vi "main_T.vi"() -> ()   [LabVIEW 2017]
uses:
  <vilib>/Platform/TimedLoop/XDataNode/timing_clust.ctl
  <vilib>/Platform/TimedLoop/XDataNode/nitl_modes.ctl
  <vilib>/Platform/TimedLoop/XDataNode/wakeup.ctl
  <vilib>/platform/TimedLoop/XDataNode/XDataNode.xnode
  <vilib>/Platform/TimedLoop/XDataNode/XDNodeRunTimeDep.lvlib
panel:
  out "Alarm Status":bool
  out "dt (ms)":u32
  in  "Tab Control":enum32{"Page 1", "Page 2"}(tab)
  in  "Pause Button 4":bool
  in  "Pause Button 3":bool
  in  "Pause Button 2":bool
  in  "Pause Button":bool
  in  "save RPM as excel":bool
  in  "save RPM as image":bool
  in  "save torque as excel":bool
  in  "save torque as image":bool
  in  "save flow as excel":bool
  in  "save flow as image":bool
  in  "save pressure as excel":bool
  in  "save press as image":bool
  out "RPM Graph":cluster{dbl[], dbl[]}(graph)
  out "t (sec)":dbl format="%#.3f"
  out "dt (sec)":dbl format="%#.3f"
  out "Torque Graph":cluster{dbl[], dbl[]}(graph)
  out "Flow Graph":cluster{dbl[], dbl[]}(graph)
  out "NI1":tag caption="NI device"
  out "Pressure Graph":cluster{dbl[], dbl[]}(graph)
  out "Turbine RPM":dbl format="%#.3f"
  out "Torque [N.m]":dbl format="%#.3f"
  out "Flow [L/min]":dbl format="%#.3f"
  out "Pressure [bar]":dbl format="%#.3f"
  out "Alarm":bool
  out "ON/OFF Pump":bool
  out "Ready / Not ready":bool
  in  "Exit":bool
  in  "Reset Chart":bool
  # "Turbine Training Unit"
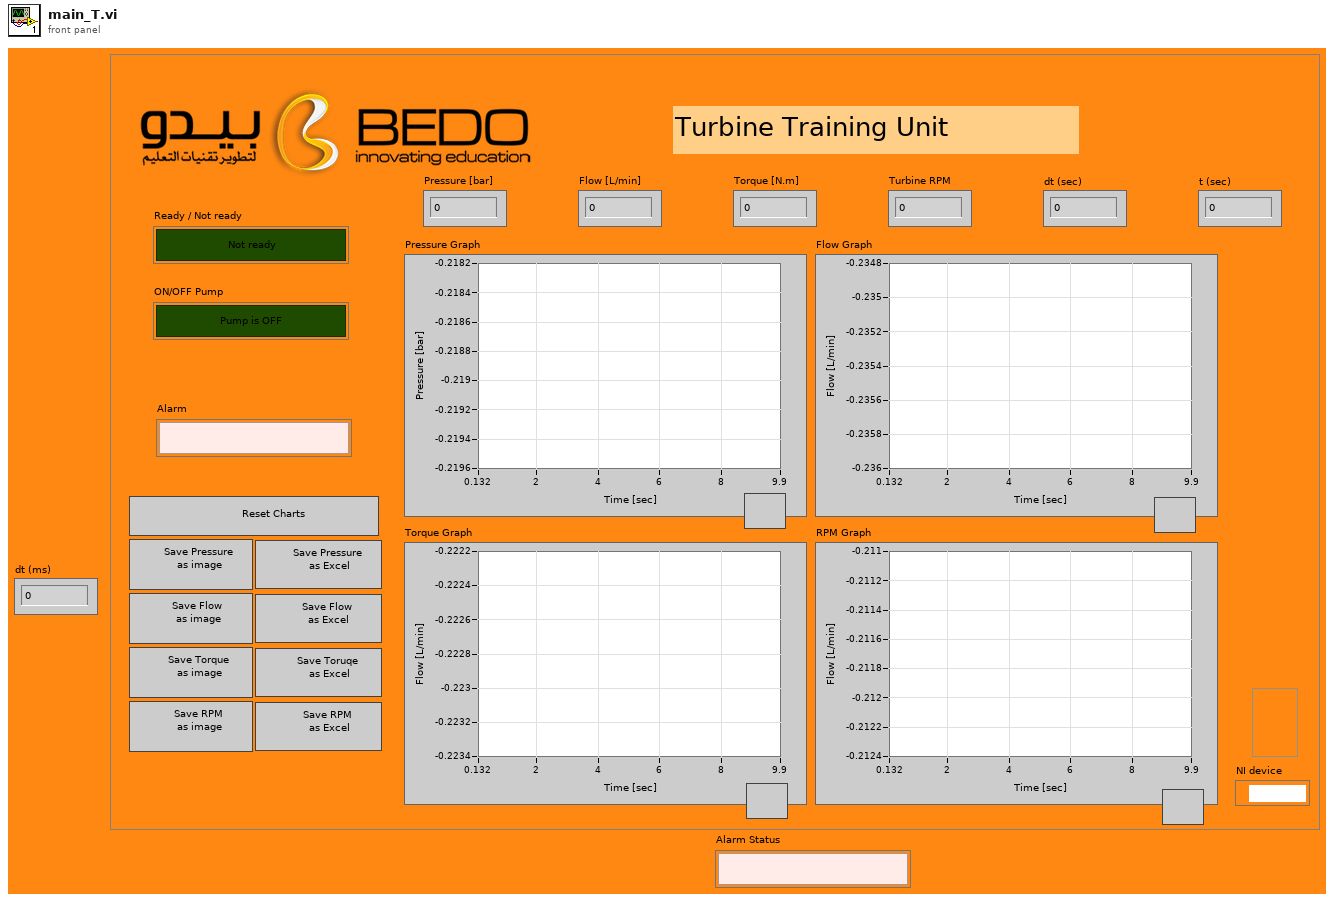
[diagram p1: front panel]
types:
  T1 = enum32{"Invalid", "Standard", "Closed", "Hidden", "Minimized", "Maximized"}
  T2 = typedef "XDNodeRunTimeDep.lvlib/timing_clust.ctl" = cluster{"Expected End [f-1]":u64, "Actual End [f-1]":u64, "Finished Late? [f-1]":bool, "Expected End [i-1]":u64, "Actual End [i-1]":u64, "Finished Late? [i-1]":bool, "Expected Start [i]":u64, "Actual Start [i]":u64, "Expected Start [f]":u64, "Actual Start [f]":u64, "Source Name":string, "Structure Name":string, "Period":i64, "Deadline":i64, "Offset":i64, "Start":i64, "Priority":i32, "Timeout":i32, "Mode":T3, "Wakeup Reason":T4, "Error":errorcluster, "Source Type":string, "Secondary Source Type":string, "Global End Time":u64, "Global Start Time":u64, "Frame Duration":u64, "Iteration Duration":u64, "Assigned CPU":i32, "I/O Scan Engine Mode":u32}
  T3 = typedef "XDNodeRunTimeDep.lvlib/nitl_modes.ctl" = enum32{"No Change", "Process missed periods, maintain original phase", "Discard missed periods, maintain original phase", "Process missed periods, ignore original phase", "Discard missed periods, ignore original phase"}
  T4 = typedef "XDNodeRunTimeDep.lvlib/wakeup.ctl" = enum32{"Normal", "Aborted", "Asynchronous wakeup", "Timing source error", "Timed loop error", "Timeout"}
  T5 = typedef "Sound Output Task ID.ctl" = u32
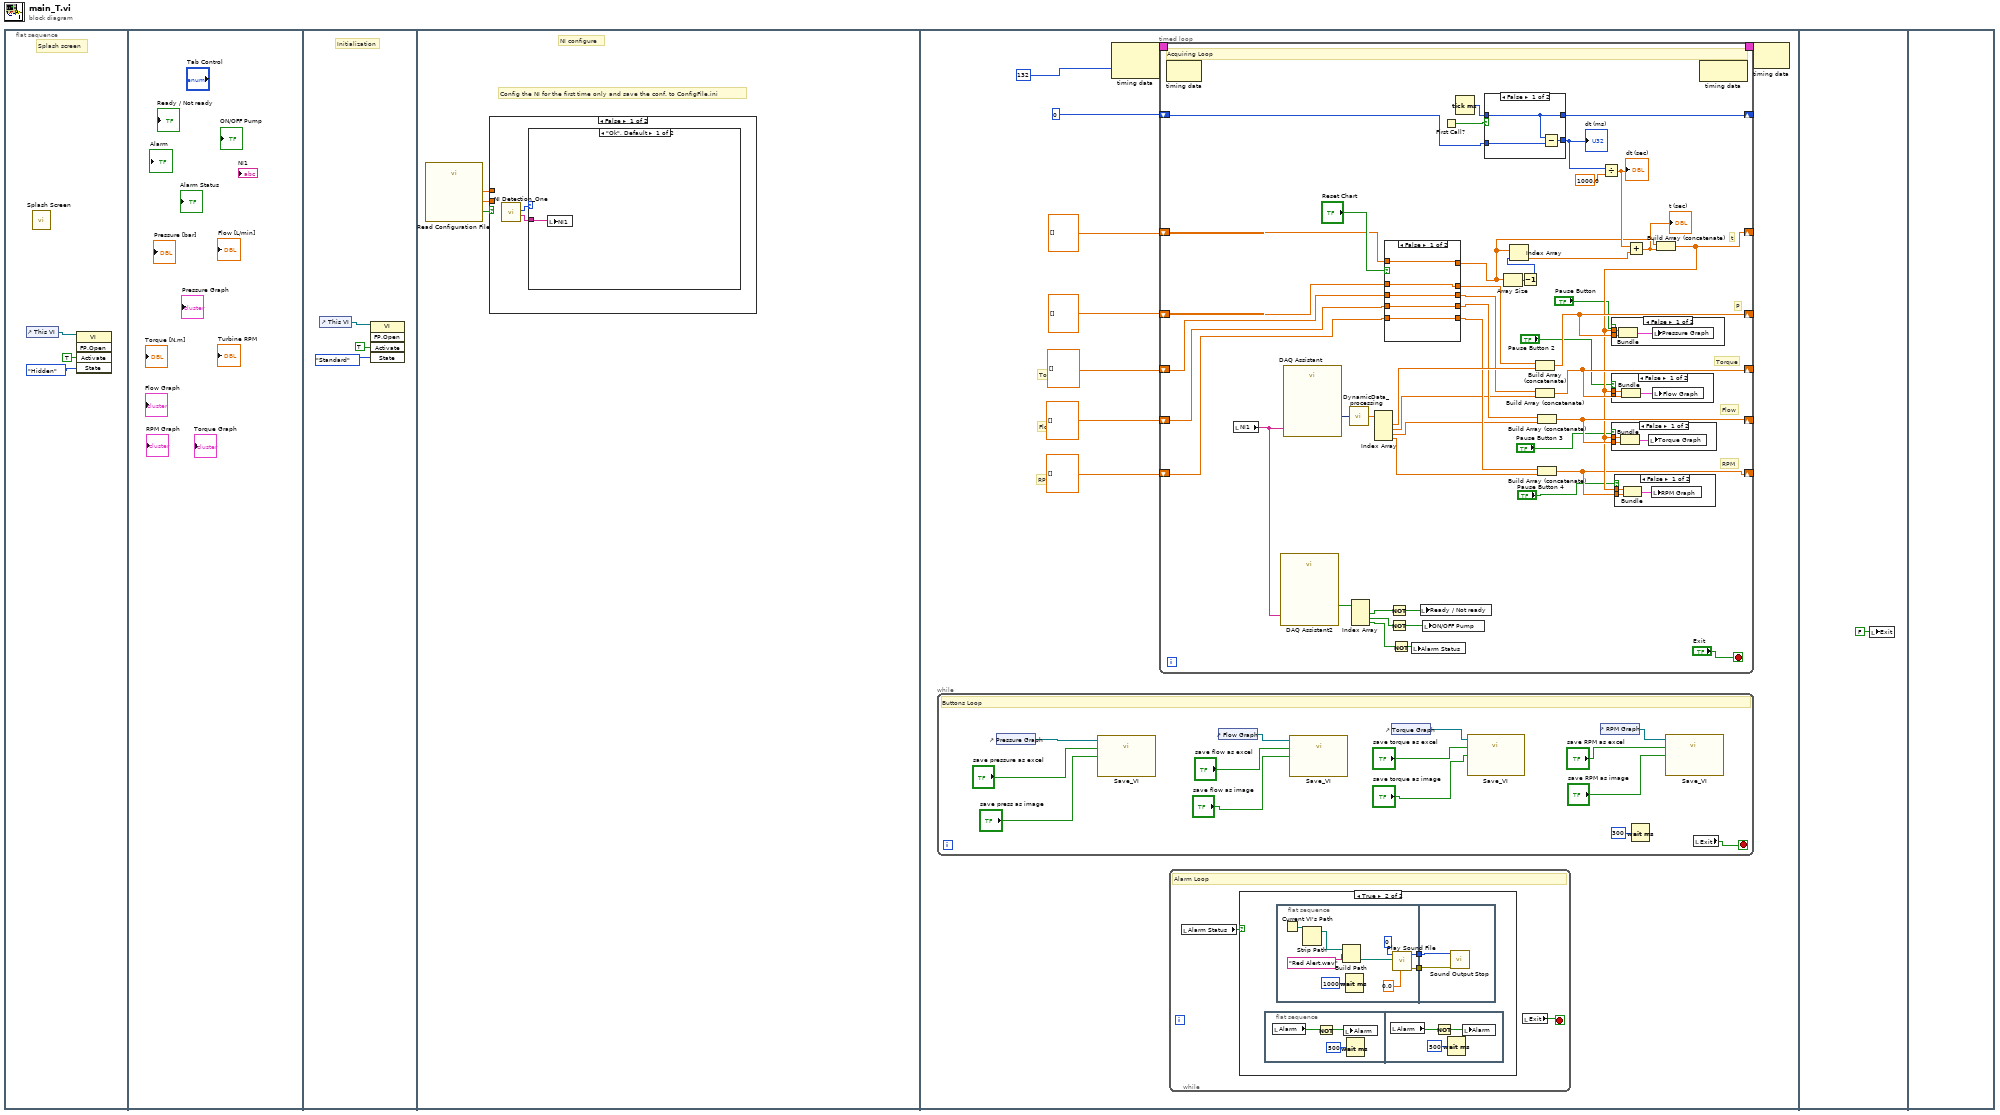
[diagram p0: block diagram]
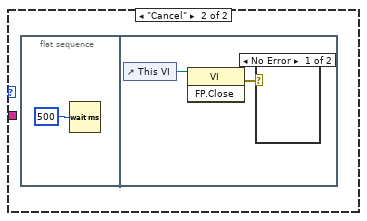
[diagram p2: hidden frame]
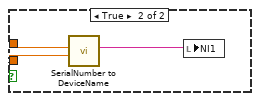
[diagram p4: hidden frame]
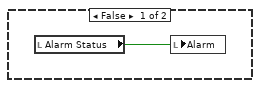
[diagram p5: hidden frame]
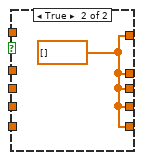
[diagram p10: hidden frame]
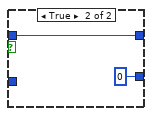
[diagram p11: hidden frame]
diagram:
  n1 = flat-sequence {
    frame #0 {
      # "Splash screen"
      n2 = control-ref of="This VI"() -> (w1:refnum<vi>)
      n3 = call "Splash Screen.vi"() -> ()  [unwired: 11 in, 1 out]
      n4 = invoke class="VI" method="FP.Open"(reference=w1, "Activate"=TRUE ("Activate?"), "State"=T1."Hidden") -> ()  [unwired: 2 in, 5 out]
    }
    frame #1 {
    }
    frame #2 {
      # "Initialization"
      n5 = control-ref of="This VI"() -> (w6:refnum<vi>)
      n6 = invoke class="VI" method="FP.Open"(reference=w6, "Activate"=TRUE ("Activate?"), "State"=T1."Standard") -> ()  [unwired: 2 in, 5 out]
    }
    frame #3 {
      # "NI configure"
      # "Config the NI for the first time only and save the conf. to ConfigFile.ini"
      n7 = call "Read Configuration File.vi"() -> ("Serial Numbers Found"=w9:bool, "NI1"=w8:dbl, "NI2"=w7:dbl)  [unwired: 13 in]
      n8 = case shown="False" w9 {
        tunnel: w8 -> [_ w18]
        tunnel: w7 -> [_ w17]
        frame False {
          n9 = call "NI Detection_One.vi"() -> ("NI 1"=w10:tag, "Ok/Cancel"=w11:enum16{"Ok", "Cancel"})  [unwired: 8 in, 1 out]
          n10 = case shown="\"Ok\", Default" w11 {
            tunnel: w10 -> [w12 _]
            frame "Ok", Default {
              n11 = local write "NI1"(w12) -> ()
            }
            frame "Cancel" {
              n12 = flat-sequence {
                frame #0 {
                  n13 = Wait (ms)(milliseconds to wait=u32 500) -> ()  [unwired: 1 out]
                }
                frame #1 {
                  n14 = control-ref of="This VI"() -> (w14:refnum<vi>)
                  n15 = invoke class="VI" method="FP.Close"(reference=w14) -> (error out=w15:errorcluster)  [unwired: 2 in, 2 out]
                  n16 = case shown="No Error" w15 {
                    frame No Error {
                    }
                    frame Error {
                    }
                  }
                }
              }
            }
          }
        }
        frame True {
          n17 = call "SerialNumber to DeviceName.vi"("NI2 Serial Number"=w17, "NI1 Serial Number"=w18) -> ("NI1 Device Name"=w16:tag)  [unwired: 8 in, 1 out]
          n18 = local write "NI1"(w16) -> ()
        }
      }
    }
    frame #4 {
      # "RPM"
      # "Flow"
      # "Torque"
      # "P"
      # "t"
      n19 = while {
        stop <- w51 stop-if-true
        # "Buttons Loop"
        n20 = control-ref of="Pressure Graph"() -> (w61:refnum<vi>)
        n21 = call "Save_VI.vi"("save press as image"="save press as image", "save pressure as excel"="save pressure as excel", "XYGraph in"=w61) -> ()  [unwired: 9 in]
        n22 = control-ref of="Flow Graph"() -> (w60:refnum<vi>)
        n23 = call "Save_VI.vi"("save press as image"="save flow as image", "save pressure as excel"="save flow as excel", "XYGraph in"=w60) -> ()  [unwired: 9 in]
        n24 = control-ref of="Torque Graph"() -> (w57:refnum<vi>)
        n25 = call "Save_VI.vi"("save press as image"="save torque as image", "save pressure as excel"="save torque as excel", "XYGraph in"=w57) -> ()  [unwired: 9 in]
        n26 = control-ref of="RPM Graph"() -> (w54:refnum<vi>)
        n27 = Wait (ms)(milliseconds to wait=u32 300) -> ()  [unwired: 1 out]
        n28 = call "Save_VI.vi"("save press as image"="save RPM as image", "save pressure as excel"="save RPM as excel", "XYGraph in"=w54) -> ()  [unwired: 9 in]
        n29 = local read "Exit"() -> (w51:bool)
      }
      n30 = node-c288(i64 132 ("Period")) -> (w27:T2)  [unwired: 1 in]
      n31 = timed-loop "Timed Loop" {
        timing: w27 -> [_]
        timing-out: [_] -> w26
        shift-right: [w105] -> _
        shift-left: u32 0 ("millisecond timer value") -> [w104]
        shift-right: [w78] -> _
        shift-left: dbl[] [] -> [w102]
        shift-right: [w82] -> _
        shift-left: dbl[] [] -> [w96]
        shift-right: [w80] -> _
        shift-left: dbl[] [] -> [w91]
        shift-right: [w79] -> _
        shift-left: dbl[] [] -> [w90]
        shift-right: [w77] -> _
        shift-left: dbl[] [] -> [w89]
        stop <- "Exit" stop-if-true
        # "RPM"
        # "Flow"
        # "Torque"
        # "P"
        # "t"
        # "Acquiring Loop"
        n32 = node-c288() -> ()  [unwired: 1 in, 1 out]
        n33 = local read "NI1"() -> (w76:tag)
        n34 = call "DAQ Assistant2"("device name"=w76) -> ("data"=w75:bool[])  [unwired: 16 in, 2 out]
        n35 = call "DAQ Assistant"("device name"=w76) -> ("data"=w95:dynamicdata)  [unwired: 16 in, 2 out]
        n36 = call "DynamicData_processing.vi"("data"=w95) -> ("DATA"=w94:dbl[])
        n37 = Index Array(array=w75) -> (element #1=w74:bool, element #2=w73:bool, element #3=w72:bool)  [unwired: 3 in]
        n38 = Index Array(array=w94) -> (element #1=w92:dbl, element #2=w85:dbl, element #3=w84:dbl, element #4=w83:dbl)  [unwired: 4 in]
        n39 = case shown="False" "Reset Chart" {
          tunnel: [w126 w127] -> w97
          tunnel: [w125 w127] -> w93
          tunnel: w102 -> [w126 _]
          tunnel: w96 -> [w125 _]
          tunnel: w91 -> [w124 _]
          tunnel: w90 -> [w123 _]
          tunnel: w89 -> [w122 _]
          tunnel: [w124 w127] -> w88
          tunnel: [w123 w127] -> w87
          tunnel: [w122 w127] -> w86
          frame False {
          }
          frame True {
            w127 = dbl[] []
          }
        }
        n40 = Not(x=w74) -> (.not. x?=w71:bool)
        n41 = Not(x=w73) -> (.not. x?=w70:bool)
        n42 = Not(x=w72) -> (.not. x?=w69:bool)
        n43 = local write "Alarm Status"(w69) -> ()
        n44 = local write "Ready / Not ready"(w71) -> ()
        n45 = local write "ON/OFF Pump"(w70) -> ()
        n46 = First Call?() -> (First Call?: T/F=w108:bool)
        n47 = Tick Count (ms)() -> (millisecond timer value=w109:u32)
        n48 = case shown="False" w108 {
          tunnel: [w128 w132] -> w105
          tunnel: w104 -> [w130 _]
          tunnel: [w129 u32 0] -> w106
          tunnel: w109 -> [w128 w132]
          frame False {
            n49 = Subtract(x=w128, y=w130) -> (x-y=w129:u32)
          }
          frame True {
          }
        }
        "dt (ms)" <- w106
        n50 = Array Size(array=w97) -> (size(s)=w101:i32)
        n51 = Decrement(x=w101) -> (x-1=w100:i32)
        n52 = Index Array(array=w97, index=w100) -> (element=w98:dbl)
        n53 = Build Array (concatenate)(w93, w92) -> (w82:dbl[])
        n54 = Build Array (concatenate)(w88, w85) -> (w80:dbl[])
        n55 = Build Array (concatenate)(w87, w84) -> (w79:dbl[])
        n56 = Build Array (concatenate)(w86, w83) -> (w77:dbl[])
        n57 = Divide(x=w106, y=1000.0) -> (x/y=w99:dbl)
        "dt (sec)" <- w99
        n58 = Add(x=w99, y=w98) -> (x+y=w64:dbl)
        "t (sec)" <- w64
        n59 = Build Array (concatenate)(w97, w64) -> (w78:dbl[])
        n60 = case shown="False" "Pause Button 2" {
          tunnel: w80 -> [w117 _]
          tunnel: w78 -> [w116 _]
          frame False {
            n61 = Bundle(w116, w117) -> (w118:cluster{dbl[], dbl[]})  [unwired: 1 in]
            n62 = local write "Flow Graph"(w118) -> ()
          }
          frame True {
          }
        }
        n63 = case shown="False" "Pause Button 3" {
          tunnel: w79 -> [w114 _]
          tunnel: w78 -> [w113 _]
          frame False {
            n64 = Bundle(w113, w114) -> (w115:cluster{dbl[], dbl[]})  [unwired: 1 in]
            n65 = local write "Torque Graph"(w115) -> ()
          }
          frame True {
          }
        }
        n66 = case shown="False" "Pause Button" {
          tunnel: w82 -> [w121 _]
          tunnel: w78 -> [w119 _]
          frame False {
            n67 = Bundle(w119, w121) -> (w120:cluster{dbl[], dbl[]})  [unwired: 1 in]
            n68 = local write "Pressure Graph"(w120) -> ()
          }
          frame True {
          }
        }
        n69 = case shown="False" "Pause Button 4" {
          tunnel: w78 -> [w111 _]
          tunnel: w77 -> [w110 _]
          frame False {
            n70 = Bundle(w111, w110) -> (w112:cluster{dbl[], dbl[]})  [unwired: 1 in]
            n71 = local write "RPM Graph"(w112) -> ()
          }
          frame True {
          }
        }
        n72 = node-c288() -> ()  [unwired: 1 in, 1 out]
      }
      n73 = while {
        stop <- w29 stop-if-true
        # "Alarm Loop"
        n74 = local read "Alarm Status"() -> (w28:bool)
        n75 = case shown="True" w28 {
          frame False {
            n76 = local read "Alarm Status"() -> (w30:bool)
            n77 = local write "Alarm"(w30) -> ()
          }
          frame True {
            n78 = flat-sequence {
              frame #0 {
                n79 = local read "Alarm"() -> (w34:bool)
                n80 = Not(x=w34) -> (.not. x?=w35:bool)
                n81 = local write "Alarm"(w35) -> ()
                n82 = Wait (ms)(milliseconds to wait=u32 500) -> ()  [unwired: 1 out]
              }
              frame #1 {
                n83 = local read "Alarm"() -> (w38:bool)
                n84 = Not(x=w38) -> (.not. x?=w37:bool)
                n85 = Wait (ms)(milliseconds to wait=u32 500) -> ()  [unwired: 1 out]
                n86 = local write "Alarm"(w37) -> ()
              }
            }
            n87 = flat-sequence {
              tunnel: [w46] -> w32
              tunnel: [w45] -> w31
              tunnel: w32 -> [w49]
              tunnel: w31 -> [w48]
              frame #0 {
                n88 = Current VI's Path() -> (path=w47:path)
                n89 = Strip Path(path=w47) -> (stripped path=w40:path)  [unwired: 1 out]
                n90 = Build Path(base path=w40, name or relative path="Red Alert.wav") -> (appended path=w42:path)
                n91 = Wait (ms)(milliseconds to wait=u32 1000) -> ()  [unwired: 1 out]
                n92 = call <vilib>:"Play Sound File.vi"("timeout (sec)"=0.0, "path"=w42, "device ID"=u32 0) -> ("error out"=w46:errorcluster, "task ID"=w45:T5)  [unwired: 7 in]
              }
              frame #1 {
                n93 = call <vilib>:"Sound Output Stop.vi"("error in (no error)"=w49, "task ID"=w48) -> ()  [unwired: 8 in, 2 out]
              }
            }
          }
        }
        n94 = local read "Exit"() -> (w29:bool)
      }
      n95 = node-c288(w26) -> ()  [unwired: 1 out]
    }
    frame #5 {
      n96 = local write "Exit"(FALSE ("Exit")) -> ()
    }
    frame #6 {
    }
  }
